vi "FVIR Status Bits Write.vi"(11 "PLC Data - FVIR Input":T1 {"Timing"."Absolute Time" format="%<%H:%M:%S%3u>t"; "Timing"."Display Time" format="%#.20f"; "Timing"."Test Time Ref" format="%#.20f"; "Timing"."Precondition Time Ref" format="%#.20f"; "Timing"."First Call Time Ref" format="%#.20f"}) -> (3 "Bit Status":string[][](array[string]))   [LabVIEW 2023]
uses:
  Modbus/Modbus FVIR Control.ctl
  Modbus/Modbus Timing.ctl
  <vilib>/Utility/miscctls.llb/LVDateTimeRec.ctl
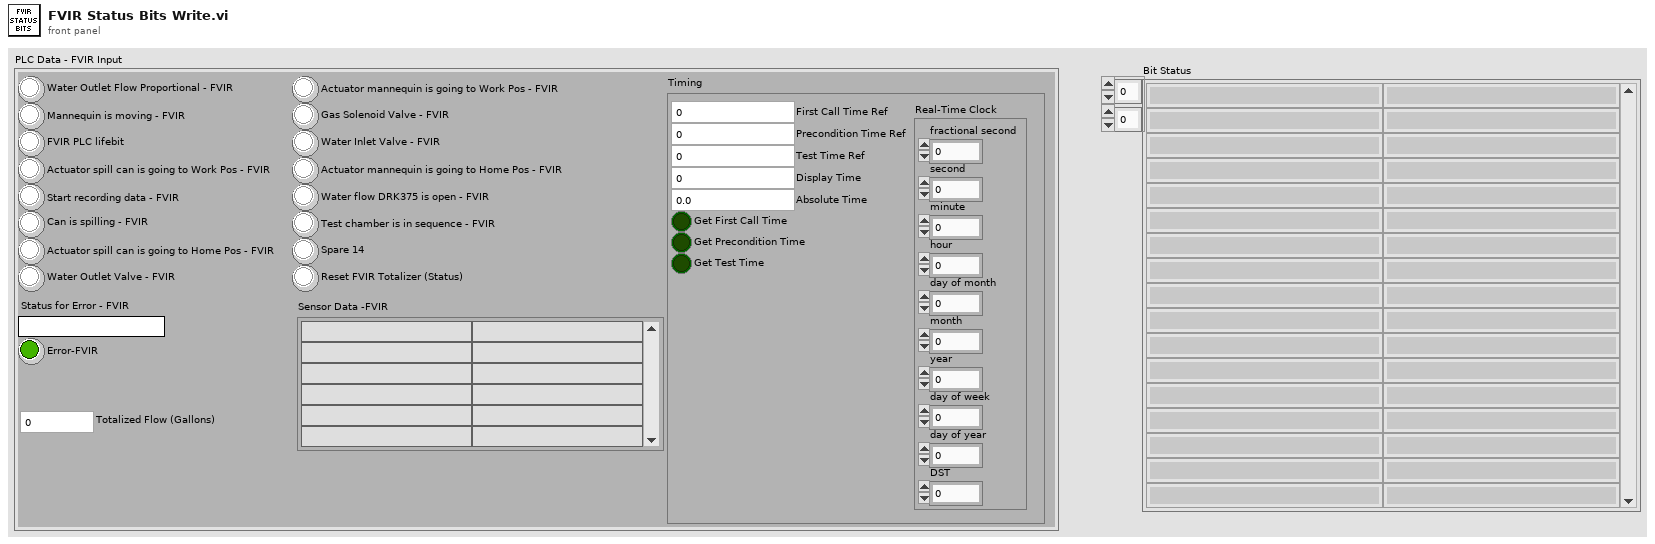
[diagram p1: front panel]
types:
  T1 = typedef "Modbus FVIR Control.ctl" = cluster{"Reset FVIR Totalizer (Status)":bool, "Spare 14":bool, "Actuator mannequin is going to Work Pos - FVIR":bool, "Actuator mannequin is going to Home Pos - FVIR":bool, "Test chamber is in sequence - FVIR ":bool, "Water flow DRK375 is open - FVIR":bool, "Gas Solenoid Valve - FVIR":bool, "Water Inlet Valve - FVIR":bool, "Water Outlet Flow Proportional - FVIR":bool, "Start recording data - FVIR":bool, "Actuator spill can is going to Work Pos - FVIR":bool, "Actuator spill can is going to Home Pos - FVIR":bool, "Water Outlet Valve - FVIR":bool, "Can is spilling - FVIR":bool, "Mannequin is moving - FVIR":bool, "FVIR PLC lifebit":bool, "Status for Error - FVIR":string, "Error-FVIR":bool, "Sensor Data -FVIR":string[][], "Totalized Flow (Gallons)":dbl, "Timing":T2}
  T2 = typedef "Modbus Timing.ctl" = cluster{"First Call Time Ref":dbl, "Precondition Time Ref":dbl, "Test Time Ref":dbl, "Get First Call Time":bool, "Get Precondition Time":bool, "Get Test Time":bool, "Display Time":dbl, "Real-Time Clock":T3, "Absolute Time":dbl}
  T3 = typedef "LVDateTimeRec.ctl" = cluster{"fractional second":dbl, "second":i32, "minute":i32, "hour":i32, "day of month":i32, "month":i32, "year":i32, "day of week":i32, "day of year":i32, "DST":i32}
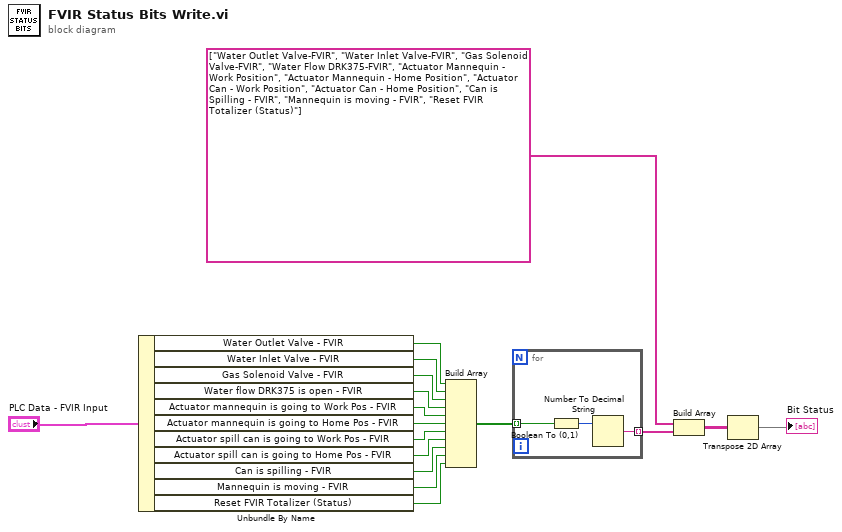
[diagram p0: block diagram]
diagram:
  n1 = Unbundle By Name("PLC Data - FVIR Input") -> ("Water Outlet Valve - FVIR"=w12:bool, "Water Inlet Valve - FVIR"=w11:bool, "Gas Solenoid Valve - FVIR"=w10:bool, "Water flow DRK375 is open - FVIR"=w9:bool, "Actuator mannequin is going to Work Pos - FVIR"=w7:bool, "Actuator mannequin is going to Home Pos - FVIR"=w6:bool, "Actuator spill can is going to Work Pos - FVIR"=w5:bool, "Actuator spill can is going to Home Pos - FVIR"=w4:bool, "Can is spilling - FVIR"=w3:bool, "Mannequin is moving - FVIR"=w2:bool, "Reset FVIR Totalizer (Status)"=w1:bool)
  n2 = Build Array(w12, w11, w10, w9, w7, w6, w5, w4, w3, w2, w1) -> (w13:bool[])
  n3 = for {
    tunnel: w13 -> [w19] mode=indexing
    tunnel: [w18] -> w14 mode=indexing
    n4 = Boolean To (0,1)(Boolean=w19) -> (0, 1=w20:i16)
    n5 = Number To Decimal String(number=w20) -> (decimal integer string=w18:string)  [unwired: 1 in]
  }
  n6 = Build Array(string[] ["Water Outlet Valve-FVIR", "Water Inlet Valve-FVIR", "Gas Solenoid Valve-FVIR", "Water Flow DRK375-FVIR", "Actuator Mannequin - Work Position", "Actuator Mannequin - Home Position", "Actuator Can - Work Position", "Actuator Can - Home Position", "Can is Spilling - FVIR", "Mannequin is moving - FVIR", "Reset FVIR Totalizer (Status)"], w14) -> (w15:string[][])
  n7 = Transpose 2D Array(2D array=w15) -> (transposed array=→"Bit Status":string[][])
